vi "init.vi"(8 "error in (no error)":errorcluster, 11 "ApplicationTC in":refnum<class "ApplicationTC.lvclass">) -> (0 "error out":errorcluster, 3 "ApplicationTC out":refnum<class "ApplicationTC.lvclass">)   [LabVIEW 2013, in "ApplicationTC.lvclass"]
uses:
  ApplicationTC.lvclass
  <userlib>/Common/Component/Application/Configuration/Application.ctl
  <userlib>/Common/Component/Application/Application/Application.lvclass/Application.ctl
  <userlib>/Common/Component/Application/Application.lvlib
  ConfigurationThisComponent/ConfigurationThisComponent.lvclass
  <userlib>/Common/Component/Application/Application/Application.lvclass
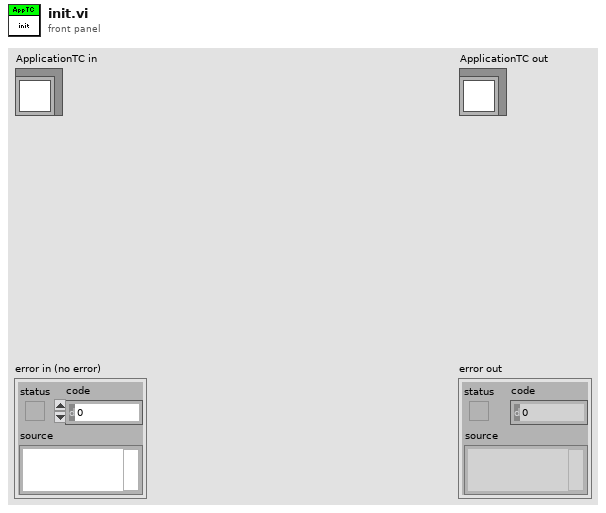
[diagram p1: front panel]
types:
  T1 = typedef "Application.lvlib/Application.ctl" = cluster{"Loop Period (ms)":u16}
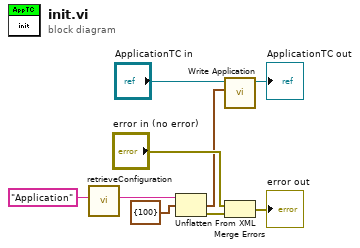
[diagram p0: block diagram]
diagram:
  n1 = call "retrieveConfiguration.vi"("configName"="Application") -> ("xmlConfig"=w6:string)  [unwired: 8 in, 2 out]
  n2 = Unflatten From XML(xml string=w6, type=T1 {"Loop Period (ms)"=100} ("Application Timing")) -> (value=w2:T1, error out=w8:errorcluster)  [unwired: 1 in]
  n3 = call <userlib>:"Write Application.vi"("Application"=w2, "Application in"="ApplicationTC in") -> ("Application out"=→"ApplicationTC out":refnum<class "ApplicationTC.lvclass">)  [unwired: 9 in]
  n4 = Merge Errors("error in (no error)", w8) -> (→"error out":errorcluster)
